vi "MTI.vi"(11 "MTI":T2(array[cluster])) -> (2 "MTI":T1[][](array[typedef]), 3 "F_z":dbl[](array[numeric]))   [LabVIEW 2019]
uses:
  Typedefs/Freq_Amp.ctl
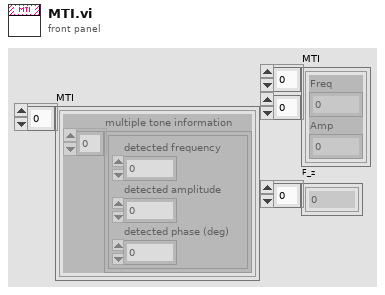
[diagram p1: front panel]
types:
  T1 = typedef "Freq_Amp.ctl" = cluster{"Freq":dbl, "Amp":dbl}
  T2 = cluster{"multiple tone information":cluster{"detected frequency":dbl, "detected amplitude":dbl, "detected phase (deg)":dbl}[]}[]
  T3 = cluster{"detected frequency":dbl, "detected amplitude":dbl, "detected phase (deg)":dbl}[]
  T4 = cluster{"detected frequency":dbl, "detected amplitude":dbl, "detected phase (deg)":dbl}
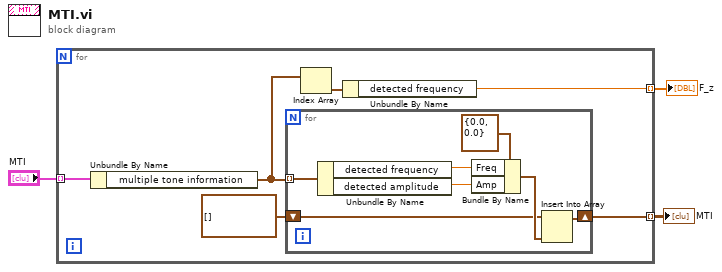
[diagram p0: block diagram]
diagram:
  n1 = for {
    tunnel: "MTI" -> [w9] mode=indexing
    tunnel: [w7] -> w2 mode=indexing
    tunnel: [w4] -> w1 mode=indexing
    n2 = Unbundle By Name(w9) -> ("multiple tone information"=w6:T3)
    n3 = for {
      tunnel: w6 -> [w16] mode=indexing
      shift-right: [w11] -> w7
      shift-left: T1[] [] -> [w10]
      n4 = Unbundle By Name(w16) -> ("detected frequency"=w14:dbl, "detected amplitude"=w13:dbl)
      n5 = Bundle By Name(cluster=T1 {"Freq"=0.0, "Amp"=0.0}, "Freq"=w14, "Amp"=w13) -> (w12:T1)
      n6 = Insert Into Array(array=w10, new element=w12) -> (w11:T1[])  [unwired: 1 in]
    }
    n7 = Index Array(array=w6) -> (element=w5:T4)  [unwired: 1 in]
    n8 = Unbundle By Name(w5) -> ("detected frequency"=w4:dbl)
  }
  "MTI" <- w2
  "F_z" <- w1
